vi "VM.vi"(0 "States":refnum<vi>, 1 "algOutputMsgs":refnum<vi>, 3 "INP":refnum<vi>, 4 "PORTS":refnum<vi>, 5 "OUTP":refnum<vi>, 6 "verifier2GUIOutputMsgs":refnum<vi>, 9 "INPUT VARS":refnum<vi>, 10 "Processes":refnum<vi>, 11 "CA2GUI":refnum<vi>, 12 "verifier2scenariousControlOutMsgs":refnum<vi>, 13 "VM2SCM":refnum<vi>, 14 "VM2GUI":refnum<vi>, 15 "VMStates":refnum<vi>) -> ()   [LabVIEW 2010]
panel:
  out "Входные  сообщения от АУ:":T1(array[cluster])
  out "Value":u32[](array[numeric])
  out "Veriphication results tbl":string[][](table) caption="Результат верификации:"
  in  "Cluster":T2
  out "Array Ports Appended array":i8[](array[numeric])
  out "Выходные  сообщения для БУС:":T1(array[cluster])
  in  "OUT Ports Array 2":cluster{"Порт":string, "Значение":bool[]}[](array[cluster]) caption="Значения входных портов:"
  out "Значение:":string[](array[string])
  out "Тип:":string[](array[string])
  out "Входные:":string[](array[string])
  out "Состояния процессов:":string[][](table)
  # "Блок верификации"
  # "Глобальные переменные"
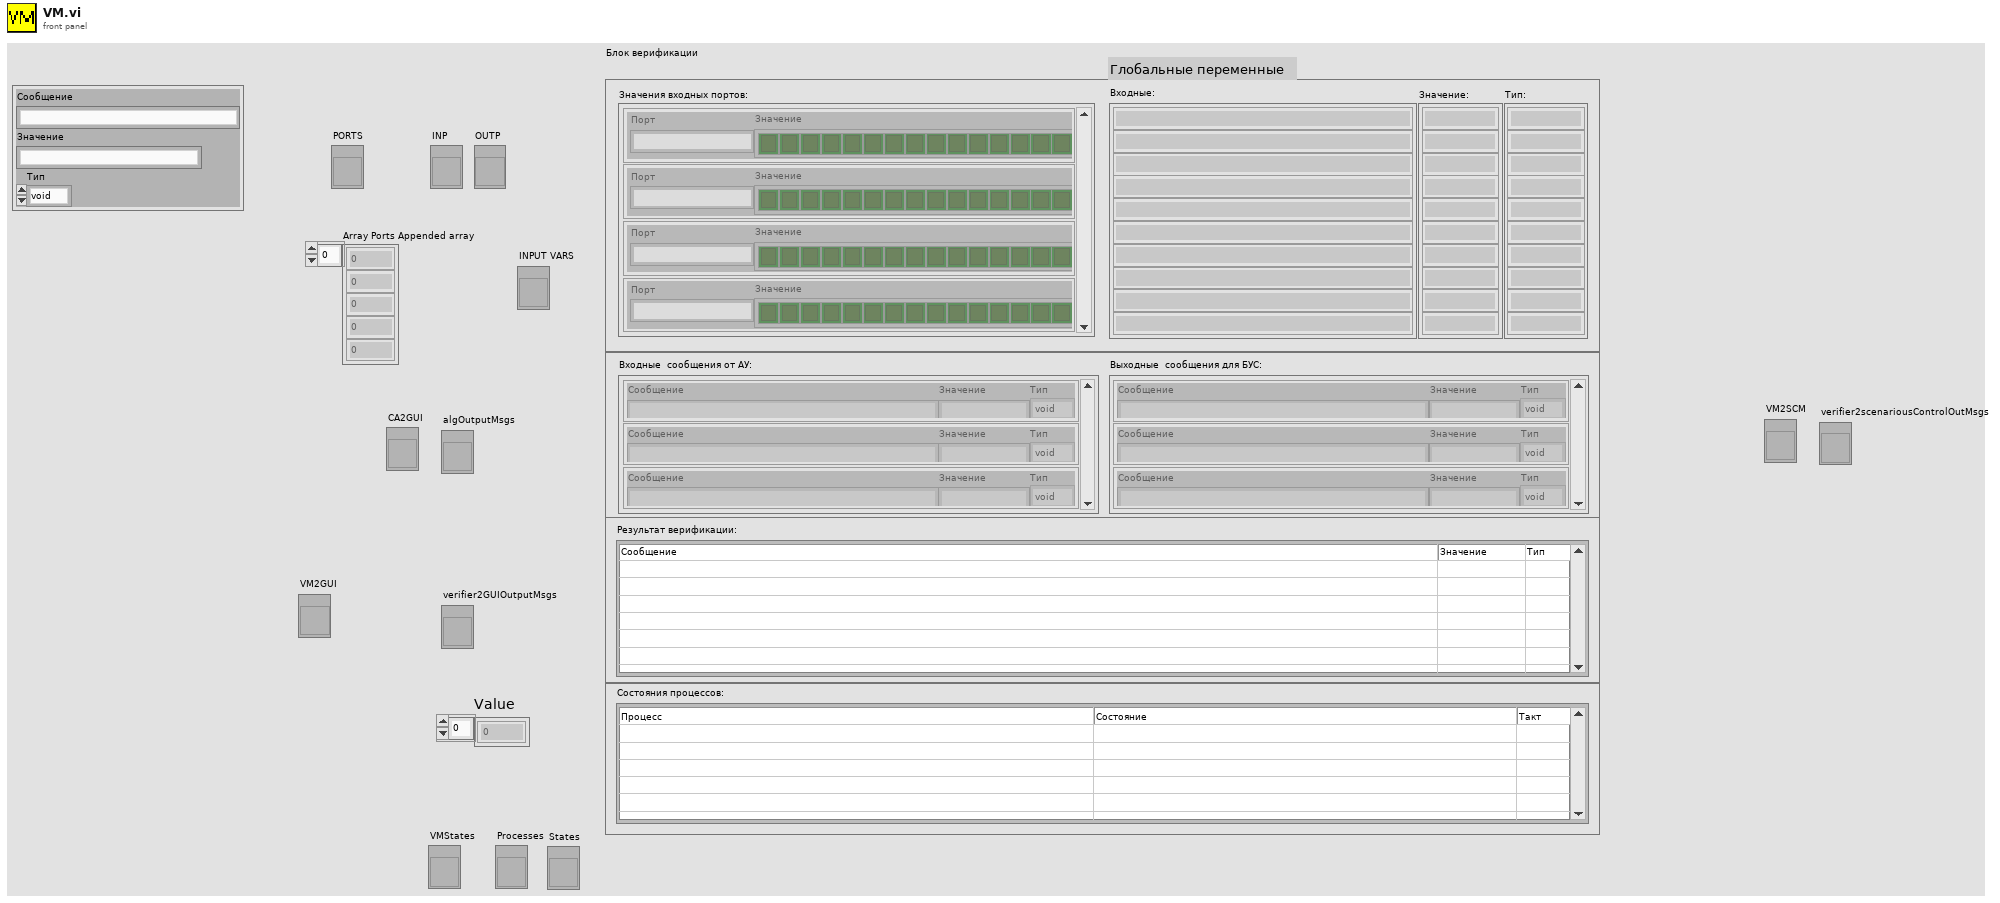
[diagram p1: front panel]
types:
  T1 = cluster{"Сообщение":string, "Значение":string, "Тип":enum16{"void", "byte", "int", "float"}}[]
  T2 = cluster{"Сообщение":string, "Значение":string, "Тип":enum16{"void", "byte", "int", "float"}}
  T3 = cluster{"Input varables names":string[], "Input varables type":string[], "Input varables ports":i32[], "Input varables bytes":i32[]}
  T4 = cluster{"Input Numbers":i32[], "Input Names":string[], "Output Names ":string[]}
  T5 = cluster{"MSG":i16, "param":i32, "Type":enum16{"void", "byte", "int", "float"}}[]
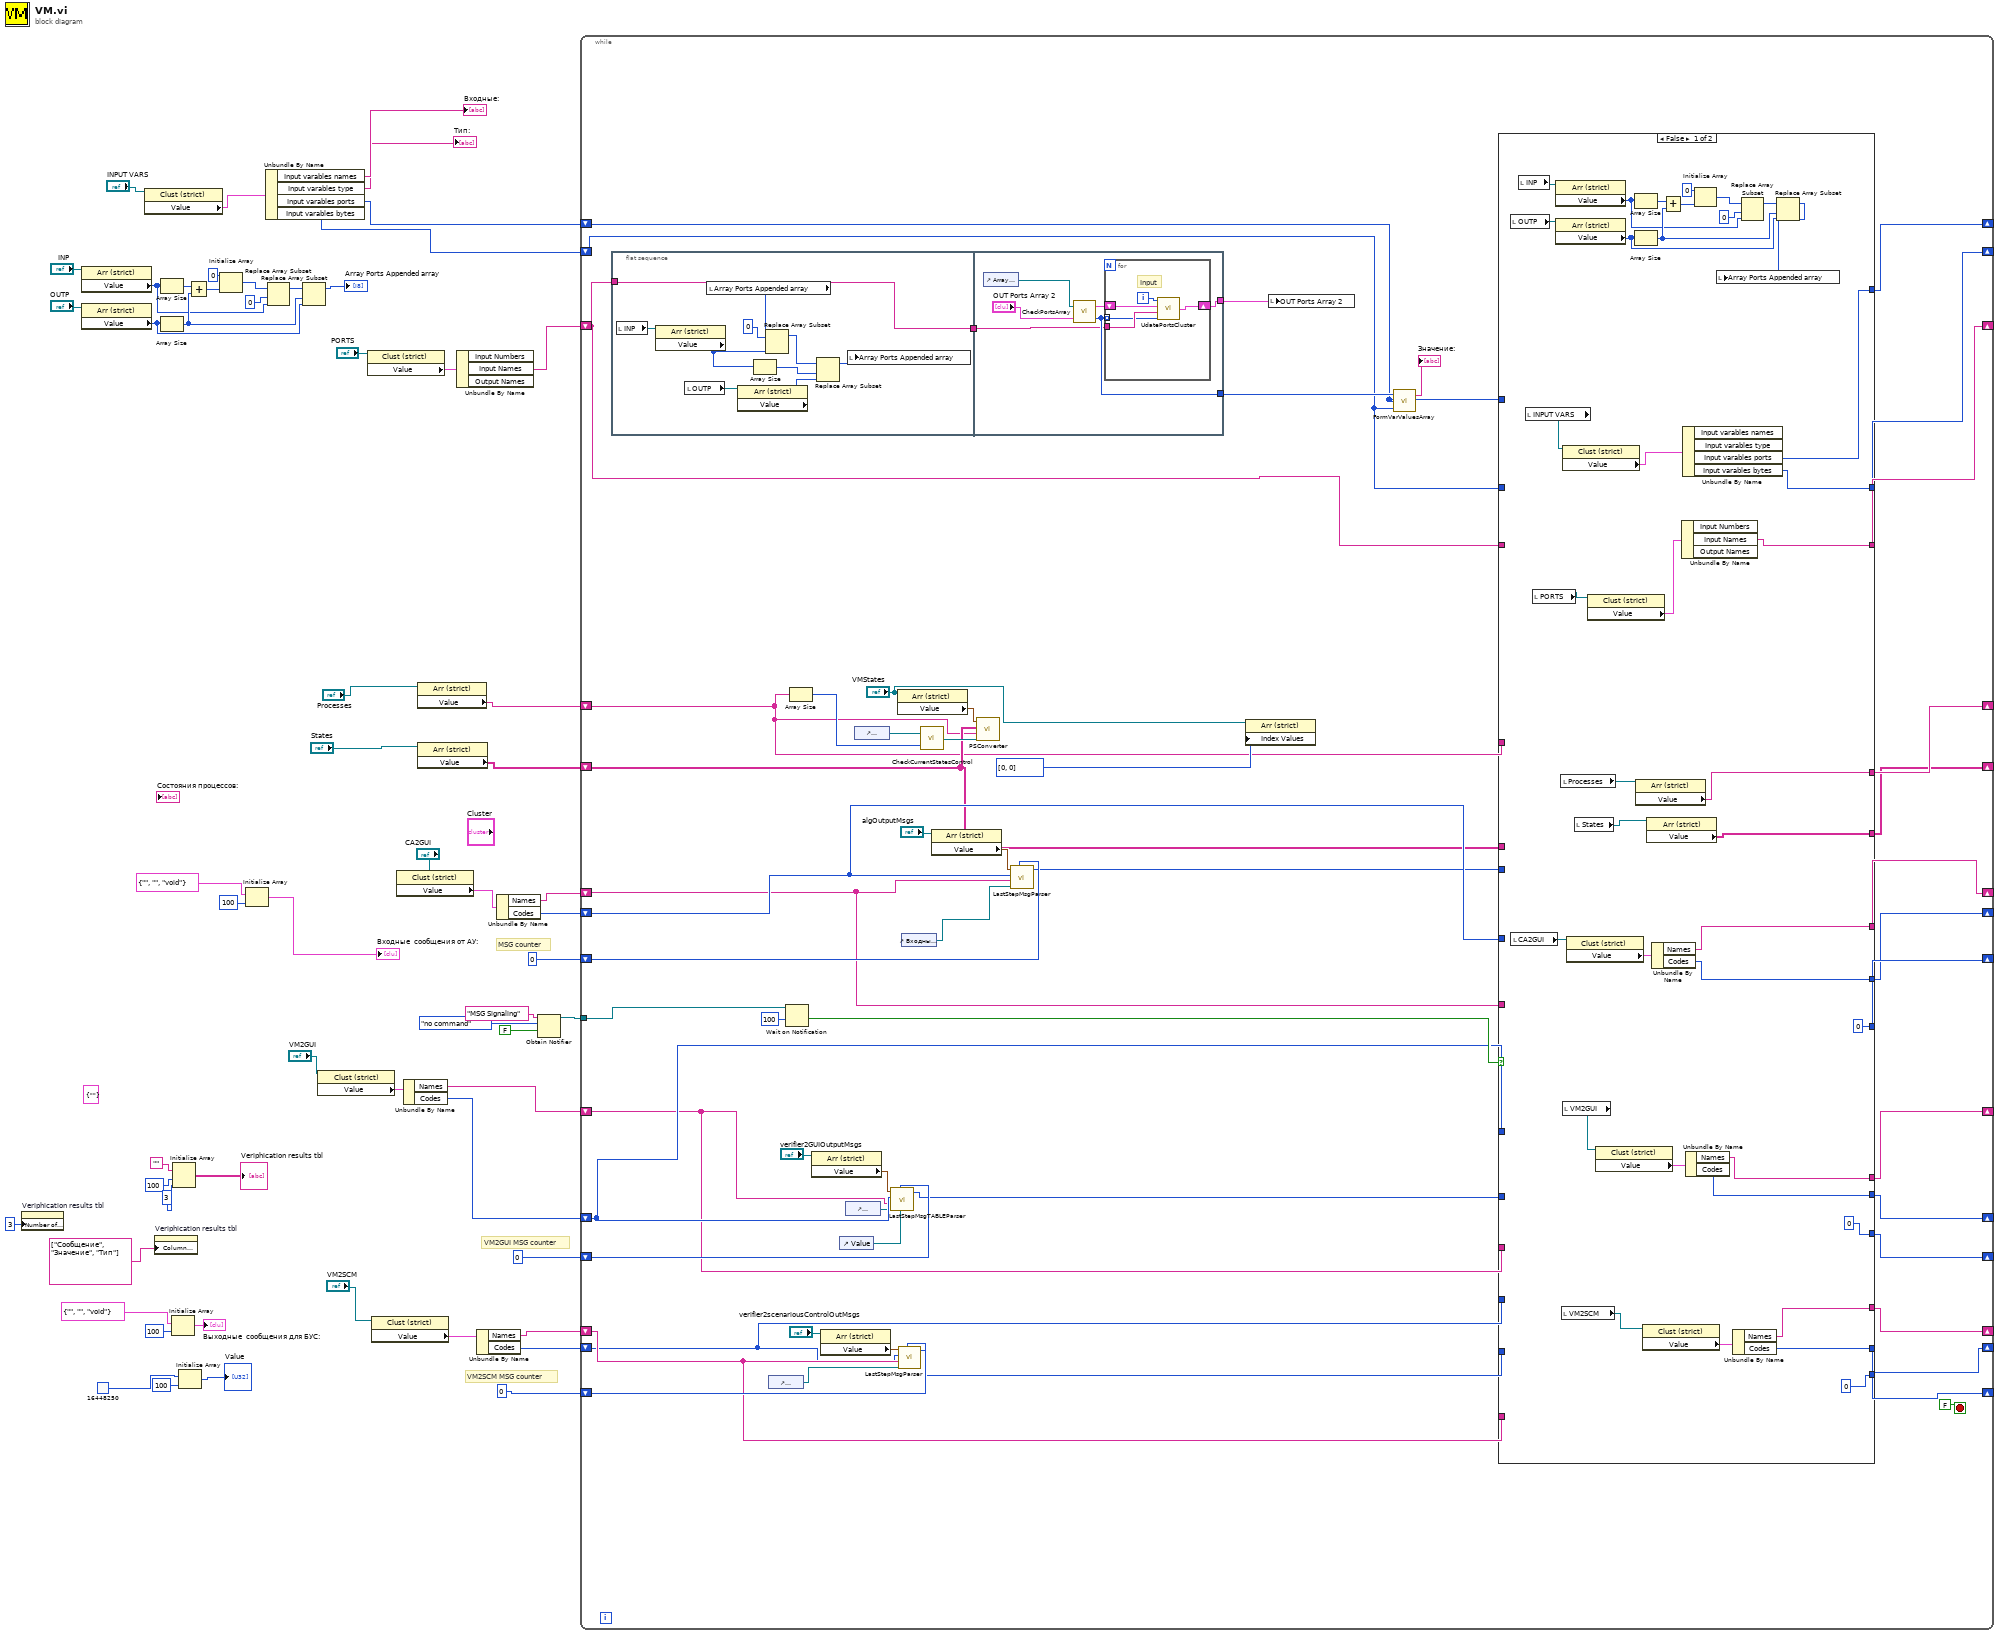
[diagram p0: block diagram]
diagram:
  (unwired) cluster{"Сообщение":string} {"Сообщение"=""} ("Cluster")
  # "VM2SCM MSG counter"
  # "VM2GUI MSG counter"
  # "MSG counter"
  n1 = property on="Veriphication results tbl" class="Tbl (strict)"("Number of Columns"=u32 3) -> ()  [unwired: 2 in, 2 out]
  n2 = property class="Arr (strict)"(reference="INP") -> ("Value"=w25:i8[])  [unwired: 1 in, 2 out]
  n3 = property class="Arr (strict)"(reference="OUTP") -> ("Value"=w24:i8[])  [unwired: 1 in, 2 out]
  n4 = property class="Clust (strict)"(reference="INPUT VARS") -> ("Value"=w46:T3)  [unwired: 1 in, 2 out]
  n5 = property on="Veriphication results tbl" class="Tbl (strict)"("Column Headers[]"=string[] ["Сообщение", "Значение", "Тип"] ("Column Header Strings[]")) -> ()  [unwired: 2 in, 2 out]
  n6 = Array Size(array=w25) -> (size(s)=w30:i32)
  n7 = Array Size(array=w24) -> (size(s)=w27:i32)
  n8 = Initialize Array(T2 {"Сообщение"="", "Значение"="", "Тип"=enum."void"} ("Cluster"), 100 ("dimension size")) -> (→"Выходные  сообщения для БУС:":T1)
  n9 = Initialize Array("", 100 ("dimension size"), 3 ("dimension size")) -> (→"Veriphication results tbl":string[][])
  n10 = Initialize Array(u32 16448250 ("Success"), 100 ("dimension size")) -> (→"Value":u32[])
  n11 = Add(x=w30, y=w27) -> (x+y=w31:i32)
  n12 = Initialize Array(i8 0 ("Numeric"), w31) -> (w29:i8[])
  n13 = Initialize Array(T2 {"Сообщение"="", "Значение"="", "Тип"=enum."void"} ("Cluster"), 100 ("dimension size")) -> (→"Входные  сообщения от АУ:":T1)
  n14 = Unbundle By Name(w46) -> ("Input varables names"=→"Входные:":string[], "Input varables type"=→"Тип:":string[], "Input varables ports"=w45:i32[], "Input varables bytes"=w44:i32[])
  n15 = Replace Array Subset(array=w29, new element=w25, index=0) -> (w26:i8[])
  n16 = Replace Array Subset(array=w26, new element=w24, index=w27) -> (→"Array Ports Appended array":i8[])
  n17 = property class="Clust (strict)"(reference="VM2GUI") -> ("Value"=w20:cluster{"Names":string[], "Codes":i32[]})  [unwired: 1 in, 2 out]
  n18 = property class="Clust (strict)"(reference="PORTS") -> ("Value"=w22:T4)  [unwired: 1 in, 2 out]
  n19 = property class="Clust (strict)"(reference="VM2SCM") -> ("Value"=w15:cluster{"Names":string[], "Codes":i32[]})  [unwired: 1 in, 2 out]
  n20 = property class="Clust (strict)"(reference="CA2GUI") -> ("Value"=w53:cluster{"Names":string[], "Codes":i32[]})  [unwired: 1 in, 2 out]
  n21 = Unbundle By Name(w20) -> ("Names"=w18:string[], "Codes"=w17:i32[])
  n22 = property class="Arr (strict)"(reference="Processes") -> ("Value"=w56:string[])  [unwired: 1 in, 2 out]
  n23 = property class="Arr (strict)"(reference="States") -> ("Value"=w55:string[][])  [unwired: 1 in, 2 out]
  n24 = Unbundle By Name(w22) -> ("Input Names"=w21:string[])  [unwired: 2 out]
  n25 = Unbundle By Name(w15) -> ("Names"=w13:string[], "Codes"=w12:i32[])
  n26 = Unbundle By Name(w53) -> ("Names"=w52:string[], "Codes"=w51:i32[])
  n27 = Obtain Notifier(name (unnamed)="MSG Signaling", notification data type=enum16{"no command", "refresh"}."no command", create if not found? (T)=FALSE) -> (notifier out=w38:refnum<notifier>)  [unwired: 1 in, 2 out]
  n28 = while {
    shift-right: [w100] -> _
    shift-left: 0 ("dimension size") -> [w106]
    tunnel: w38 -> [w103]
    shift-right: [w98] -> _
    shift-left: w51 -> [w99]
    shift-right: [w97] -> _
    shift-left: w52 -> [w96]
    shift-right: [w91] -> _
    shift-left: w55 -> [w94]
    shift-right: [w92] -> _
    shift-left: w56 -> [w93]
    shift-right: [w85] -> _
    shift-left: w44 -> [w89]
    shift-right: [w86] -> _
    shift-left: w45 -> [w90]
    shift-right: [w87] -> _
    shift-left: w21 -> [w88]
    shift-right: [w80] -> _
    shift-left: w18 -> [w64]
    shift-right: [w79] -> _
    shift-left: w17 -> [w65]
    shift-right: [w78] -> _
    shift-left: 0 ("dimension size") -> [w67]
    shift-right: [w70] -> _
    shift-left: w13 -> [w72]
    shift-right: [w69] -> _
    shift-left: w12 -> [w71]
    shift-right: [w68] -> _
    shift-left: 0 ("dimension size") -> [w74]
    stop <- FALSE ("stop") stop-if-true
    n29 = flat-sequence {
      tunnel: w88 -> [w124]
      tunnel: [w124] -> w82
      tunnel: [w129] -> w105
      tunnel: [w126] -> w83
      tunnel: w82 -> [w128]
      frame #0 {
        n30 = local read "INP"() -> (w115:refnum<vi>)
        n31 = property class="Arr (strict)"(reference=w115) -> ("Value"=w123:i8[])  [unwired: 1 in, 2 out]
        n32 = local read "OUTP"() -> (w116:refnum<vi>)
        n33 = local read "Array Ports Appended array"() -> (w120:i8[])
        n34 = property class="Arr (strict)"(reference=w116) -> ("Value"=w122:i8[])  [unwired: 1 in, 2 out]
        n35 = Array Size(array=w123) -> (size(s)=w119:i32)
        n36 = Replace Array Subset(array=w120, new element=w123, index=0) -> (w118:i8[])
        n37 = Replace Array Subset(array=w118, new element=w122, index=w119) -> (w121:i8[])
        n38 = local write "Array Ports Appended array"(w121) -> ()
      }
      frame #1 {
        n39 = control-ref of="Array Ports Appended array"() -> (w125:refnum<vi>)
        n40 = call "CheckPortsArray.vi"("INP Ports Array 2"="OUT Ports Array 2", "INP"=w125) -> ("Value"=w129:i8[], "INP Ports Array"=w130:cluster{"String":string, "Array 2":bool[]}[])
        n41 = for {
          tunnel: w129 -> [w134] mode=indexing
          tunnel: w128 -> [w135]
          shift-right: [w131] -> w126
          shift-left: w130 -> [w132]
          i -> [w133]
          # "Input"
          n42 = call "UdatePortsCluster.vi"("Numeric 2"=w134, "Input Names"=w135, "Ports Array"=w132, "index"=w133) -> ("INP Ports Array 2"=w131:cluster{"String":string, "Array 2":bool[]}[])
        }
      }
    }
    n43 = control-ref of="Выходные  сообщения для БУС:"() -> (w75:refnum<vi>)
    n44 = Wait on Notification(notifier=w103, timeout in ms (-1)=100) -> (timed out?=w102:bool)  [unwired: 2 in, 3 out]
    n45 = Array Size(array=w93) -> (size(s)=w95:i32)
    n46 = property class="Arr (strict)"(reference="verifier2GUIOutputMsgs") -> ("Value"=w66:cluster{"MSG":i16, "param":i32, "Type":i16}[])  [unwired: 1 in, 2 out]
    n47 = property class="Arr (strict)"(reference="verifier2scenariousControlOutMsgs") -> ("Value"=w77:cluster{"MSG":i16, "param":i32, "Type":i16}[])  [unwired: 1 in, 2 out]
    n48 = control-ref of="Value"() -> (w61:refnum<vi>)
    n49 = control-ref of="Veriphication results tbl"() -> (w63:refnum<vi>)
    n50 = control-ref of="Состояния процессов:"() -> (w113:refnum<vi>)
    n51 = call "LastStepMsgTABLEParser.vi"("Color Arr Refnum"=w61, "Tbl Refnum"=w63, "Out MSG Names"=w64, "old msg counter"=w67, "Codes"=w65, "Msg Array"=w66) -> ("current msg counter"=w62:i32)  [unwired: 3 in, 1 out]
    n52 = property class="Arr (strict)"(reference="VMStates") -> ("Value"=w114:cluster{"TimeInState":u16, "cur_state":i8}[])  [unwired: 1 in, 2 out]
    n53 = call "LastStepMsgParser.vi"("Arr Refnum"=w75, "Out MSG Names"=w72, "old msg counter"=w74, "Codes"=w71, "Msg Array"=w77) -> ("current msg counter"=w73:i32)  [unwired: 4 in, 1 out]
    n54 = control-ref of="Входные  сообщения от АУ:"() -> (w60:refnum<vi>)
    n55 = call "CheckCurrentStatesControl.vi"("Processes"=w95, "Inp reference"=w113) -> ("Out Refnum"=w112:refnum<vi>)
    n56 = property class="Arr (strict)"(reference="algOutputMsgs") -> ("Value"=w107:T5)  [unwired: 1 in, 2 out]
    n57 = call "PSConverter.vi"("Tbl Refnum"=w112, "PROC"=w93, "STATES"=w94, "Input claster"=w114) -> ()  [unwired: 1 out]
    n58 = call "LastStepMsgParser.vi"("Arr Refnum"=w60, "Out MSG Names"=w96, "old msg counter"=w106, "Codes"=w99, "Msg Array"=w107) -> ("current msg counter"=w101:i32)  [unwired: 4 in, 1 out]
    n59 = property class="Arr (strict)"(reference="VMStates", "Index Values"=u32[] [0, 0]) -> ()  [unwired: 1 in, 2 out]
    n60 = local write "OUT Ports Array 2"(w83) -> ()
    n61 = call "FormVarValuesArray.vi"("varables bytes"=w89, "varables ports"=w90, "Ports"=w105) -> ("Values Array"=→"Значение:":string[])  [unwired: 1 in]
    n62 = case shown="False" w102 {
      tunnel: w101 -> [_ w185]
      tunnel: [0 ("current msg counter") w185] -> w100
      tunnel: w99 -> [_ w187]
      tunnel: [w169 w187] -> w98
      tunnel: [w170 w186] -> w97
      tunnel: w96 -> [_ w186]
      tunnel: w94 -> [_ w183]
      tunnel: w93 -> [_ w184]
      tunnel: [w167 w184] -> w92
      tunnel: [w165 w183] -> w91
      tunnel: w90 -> [_ w181]
      tunnel: w89 -> [_ w180]
      tunnel: w88 -> [_ w182]
      tunnel: [w146 w182] -> w87
      tunnel: [w160 w181] -> w86
      tunnel: [w161 w180] -> w85
      tunnel: w64 -> [_ w178]
      tunnel: w62 -> [_ w179]
      tunnel: [w143 w178] -> w80
      tunnel: [w142 w174] -> w79
      tunnel: [0 ("current msg counter") w179] -> w78
      tunnel: w73 -> [_ w176]
      tunnel: w72 -> [_ w175]
      tunnel: w71 -> [_ w177]
      tunnel: [w138 w175] -> w70
      tunnel: [w137 w177] -> w69
      tunnel: [0 ("current msg counter") w176] -> w68
      tunnel: w65 -> [_ w174]
      frame False {
        n63 = local read "OUTP"() -> (w149:refnum<vi>)
        n64 = local read "CA2GUI"() -> (w172:refnum<vi>)
        n65 = local read "INP"() -> (w150:refnum<vi>)
        n66 = local read "INPUT VARS"() -> (w162:refnum<vi>)
        n67 = local read "PORTS"() -> (w164:refnum<vi>)
        n68 = property class="Arr (strict)"(reference=w150) -> ("Value"=w152:i8[])  [unwired: 1 in, 2 out]
        n69 = property class="Arr (strict)"(reference=w149) -> ("Value"=w151:i8[])  [unwired: 1 in, 2 out]
        n70 = local read "Processes"() -> (w168:refnum<vi>)
        n71 = local read "VM2SCM"() -> (w139:refnum<vi>)
        n72 = property class="Clust (strict)"(reference=w162) -> ("Value"=w163:T3)  [unwired: 1 in, 2 out]
        n73 = local read "VM2GUI"() -> (w145:refnum<vi>)
        n74 = property class="Clust (strict)"(reference=w172) -> ("Value"=w171:cluster{"Names":string[], "Codes":i32[]})  [unwired: 1 in, 2 out]
        n75 = local read "States"() -> (w166:refnum<vi>)
        n76 = property class="Clust (strict)"(reference=w164) -> ("Value"=w147:T4)  [unwired: 1 in, 2 out]
        n77 = property class="Clust (strict)"(reference=w145) -> ("Value"=w144:cluster{"Names":string[], "Codes":i32[]})  [unwired: 1 in, 2 out]
        n78 = Array Size(array=w152) -> (size(s)=w157:i32)
        n79 = Array Size(array=w151) -> (size(s)=w154:i32)
        n80 = property class="Arr (strict)"(reference=w168) -> ("Value"=w167:string[])  [unwired: 1 in, 2 out]
        n81 = property class="Clust (strict)"(reference=w139) -> ("Value"=w140:cluster{"Names":string[], "Codes":i32[]})  [unwired: 1 in, 2 out]
        n82 = property class="Arr (strict)"(reference=w166) -> ("Value"=w165:string[][])  [unwired: 1 in, 2 out]
        n83 = Unbundle By Name(w171) -> ("Names"=w170:string[], "Codes"=w169:i32[])
        n84 = Add(x=w157, y=w154) -> (x+y=w158:i32)
        n85 = Unbundle By Name(w147) -> ("Input Names"=w146:string[])  [unwired: 2 out]
        n86 = Unbundle By Name(w163) -> ("Input varables ports"=w160:i32[], "Input varables bytes"=w161:i32[])  [unwired: 2 out]
        n87 = Unbundle By Name(w144) -> ("Names"=w143:string[], "Codes"=w142:i32[])
        n88 = Initialize Array(i8 0 ("Numeric"), w158) -> (w156:i8[])
        n89 = Unbundle By Name(w140) -> ("Names"=w138:string[], "Codes"=w137:i32[])
        n90 = Replace Array Subset(array=w156, new element=w152, index=0) -> (w153:i8[])
        n91 = Replace Array Subset(array=w153, new element=w151, index=w154) -> (w148:i8[])
        n92 = local write "Array Ports Appended array"(w148) -> ()
      }
      frame True {
      }
    }
  }
